vi "Write Roles.vi"(8 "error in (no error)":errorcluster, 10 "Roles":T1, 11 "EnemyPossessionAtOurFieldPlay in":refnum<class "EnemyPossessionAtOurFieldPlay.lvclass">) -> (0 "error out":errorcluster, 3 "EnemyPossessionAtOurFieldPlay out":refnum<class "EnemyPossessionAtOurFieldPlay.lvclass">)   [LabVIEW 2020, in "EnemyPossessionAtOurFieldPlay.lvclass"]
uses:
  EnemyPossessionAtOurFieldPlay.lvclass
  EnemyPossessionAtOurFieldRoles.ctl
  ShootRole_class/ShootRole.lvclass
  MarkerRole_class/MarkerRole.lvclass
  EnemyPossessionAtOurFieldPlay.lvclass/EnemyPossessionAtOurFieldPlay.ctl
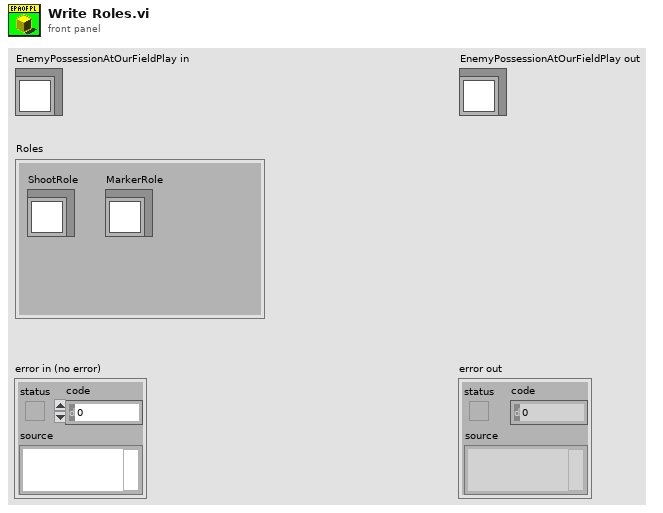
[diagram p1: front panel]
types:
  T1 = typedef "EnemyPossessionAtOurFieldRoles.ctl" = cluster{"ShootRole":refnum<class "ShootRole.lvclass">, "MarkerRole":refnum<class "MarkerRole.lvclass">}
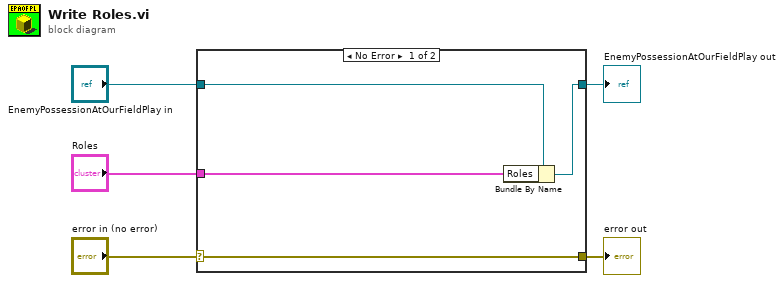
[diagram p0: block diagram]
diagram:
  n1 = case shown="No Error" "error in (no error)" {
    selector: "error in (no error)" -> [w9 w10]
    tunnel: [w9 w10] -> w4
    tunnel: [w7 w11] -> w2
    tunnel: "EnemyPossessionAtOurFieldPlay in" -> [w8 w11]
    tunnel: "Roles" -> [w6 _]
    frame No Error {
      n2 = Bundle By Name(cluster=w8, "Roles"=w6) -> (w7:refnum<class "EnemyPossessionAtOurFieldPlay.lvclass">)
    }
    frame Error {
    }
  }
  "error out" <- w4
  "EnemyPossessionAtOurFieldPlay out" <- w2
